vi "Digital_Input_16Channels.vi"(1 "IO":T1={"DI 0"="Mod1/DIO2", "DI 1"="Mod1/DIO2", "DI 2"="Mod1/DIO2", "DI 3"="Mod1/DIO2", "DI 4"="Mod1/DIO2", "DI 5"="Mod1/DIO2", "DI 6"="Mod1/DIO2", "DI 7"="Mod1/DIO2", "DI 8"="Mod1/DIO2", "DI 9"="Mod1/DIO2", "DI 10"="Mod1/DIO2", "DI 11"="Mod1/DIO2", "DI 12"="Mod1/DIO2", "DI 13"="Mod1/DIO2", "DI 14"="Mod1/DIO2", "DI 15"="Mod1/DIO2"}) -> (0 "States":bool[](array[boolean]))   [LabVIEW 2015]
uses:
  <vilib>/rvi/eio/common/nirviEmuTemplateMethod_errors.vi
  <vilib>/eio/EIONode/EIONode.xnode
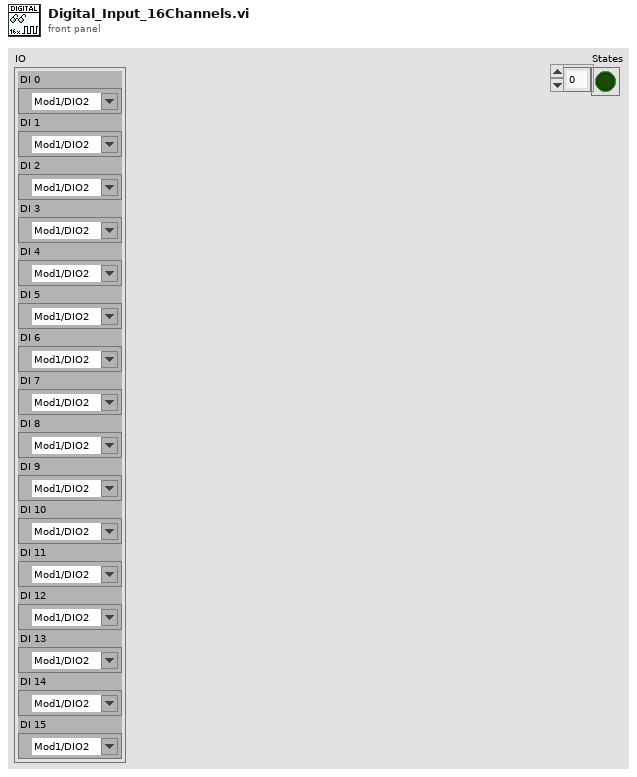
[diagram p1: front panel]
types:
  T1 = cluster{"DI 0":refnum<k21>, "DI 1":refnum<k21>, "DI 2":refnum<k21>, "DI 3":refnum<k21>, "DI 4":refnum<k21>, "DI 5":refnum<k21>, "DI 6":refnum<k21>, "DI 7":refnum<k21>, "DI 8":refnum<k21>, "DI 9":refnum<k21>, "DI 10":refnum<k21>, "DI 11":refnum<k21>, "DI 12":refnum<k21>, "DI 13":refnum<k21>, "DI 14":refnum<k21>, "DI 15":refnum<k21>}
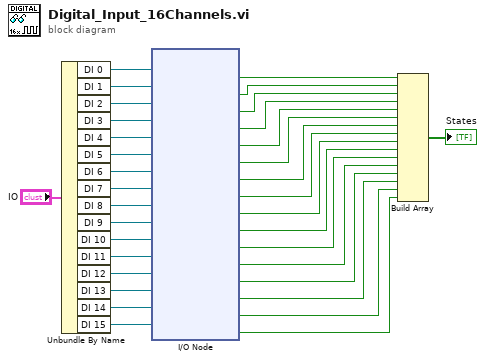
[diagram p0: block diagram]
diagram:
  n1 = Unbundle By Name("IO") -> ("DI 0"=w33:refnum<k21>, "DI 1"=w32:refnum<k21>, "DI 2"=w31:refnum<k21>, "DI 3"=w30:refnum<k21>, "DI 4"=w29:refnum<k21>, "DI 5"=w28:refnum<k21>, "DI 6"=w27:refnum<k21>, "DI 7"=w26:refnum<k21>, "DI 8"=w16:refnum<k21>, "DI 9"=w15:refnum<k21>, "DI 10"=w14:refnum<k21>, "DI 11"=w13:refnum<k21>, "DI 12"=w12:refnum<k21>, "DI 13"=w11:refnum<k21>, "DI 14"=w10:refnum<k21>, "DI 15"=w9:refnum<k21>)
  n2 = xnode "I/O Node"("FPGA I/O In"=w33, "FPGA I/O In"=w32, "FPGA I/O In"=w31, "FPGA I/O In"=w30, "FPGA I/O In"=w29, "FPGA I/O In"=w28, "FPGA I/O In"=w27, "FPGA I/O In"=w26, "FPGA I/O In"=w16, "FPGA I/O In"=w15, "FPGA I/O In"=w14, "FPGA I/O In"=w13, "FPGA I/O In"=w12, "FPGA I/O In"=w11, "FPGA I/O In"=w10, "FPGA I/O In"=w9) -> ("I/O Item"=w25:bool, "I/O Item"=w24:bool, "I/O Item"=w23:bool, "I/O Item"=w22:bool, "I/O Item"=w21:bool, "I/O Item"=w20:bool, "I/O Item"=w19:bool, "I/O Item"=w18:bool, "I/O Item"=w8:bool, "I/O Item"=w7:bool, "I/O Item"=w6:bool, "I/O Item"=w5:bool, "I/O Item"=w4:bool, "I/O Item"=w3:bool, "I/O Item"=w2:bool, "I/O Item"=w1:bool)  [unwired: 16 out]
  n3 = Build Array(w25, w24, w23, w22, w21, w20, w19, w18, w8, w7, w6, w5, w4, w3, w2, w1) -> (→"States":bool[])
